vi "rethinkdb_json_paths.vi"(8 "error in (no error)":errorcluster, 10 "args":string[](array[string]), 11 "tokens":T1[](array[typedef])) -> (0 "error out":errorcluster, 2 "value_indexes":i32[](array[numeric]), 3 "value_paths":string[](array[string]), 5 "indent":i32[](array[numeric]))   [LabVIEW 2017]
uses:
  rethinkdb_json_token.ctl
panel:
  # "a -> {\"a\":1}\na/b -> {\"a\":{\"b\":1}}\na@0 -> {\"a\":[1]}\na@0/b -> {\"a\":[{\"b\":1}]"
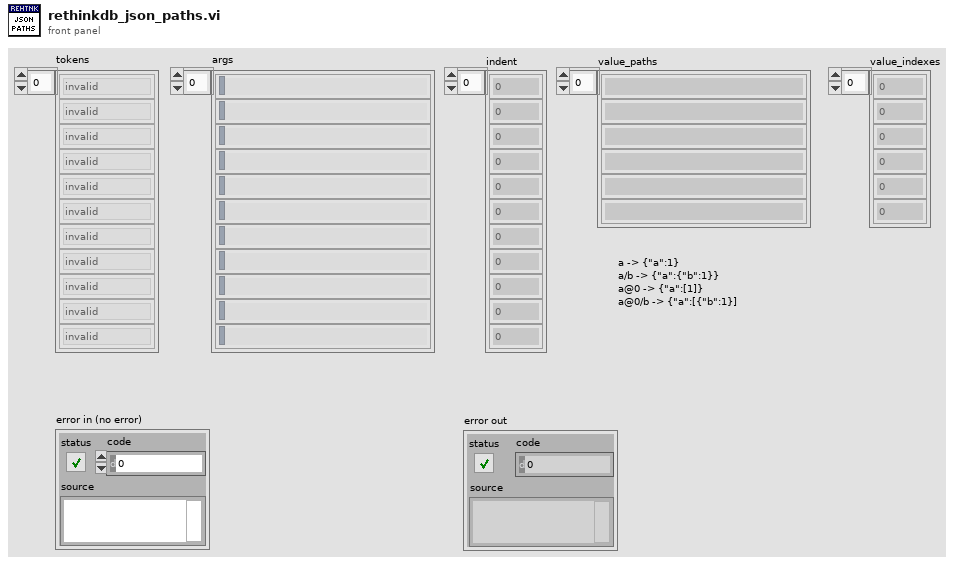
[diagram p1: front panel]
types:
  T1 = typedef "rethinkdb_json_token.ctl" = enum8{"invalid", "null", "boolean", "decimal", "float", "string", "key", "comma", "object_start", "object_end", "array_start", "array_end", "end"}
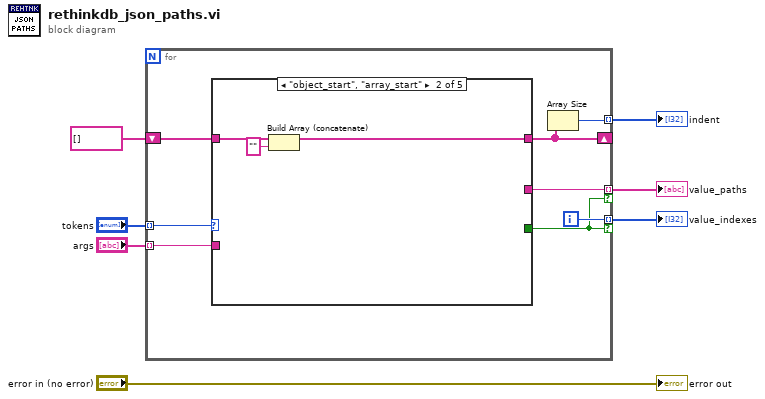
[diagram p0: block diagram]
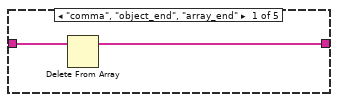
[diagram p2: hidden frame]
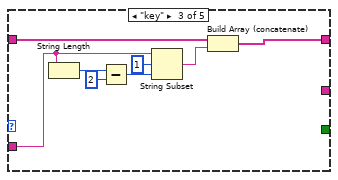
[diagram p3: hidden frame]
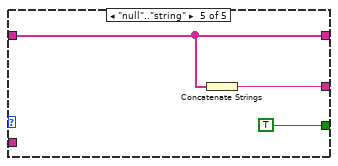
[diagram p5: hidden frame]
diagram:
  n1 = for {
    tunnel: "tokens" -> [w15] mode=indexing
    tunnel: [w12] -> w6 mode=indexing
    shift-right: [w13] -> _
    shift-left: string[] [] -> [w14]
    tunnel: "args" -> [w11] mode=indexing
    tunnel: [w10] -> w3 mode=indexing if=w8
    tunnel: [w9] -> w2 mode=indexing if=w8
    i -> [w9]
    n2 = case shown="\"object_start\", \"array_start\"" w15 {
      tunnel: [w16 w19 w27 _ w31] -> w13
      tunnel: w14 -> [w17 w20 w28 _ w31]
      tunnel: w11 -> [_ _ w22 _ _]
      tunnel: [_ _ _ _ w30] -> w10
      tunnel: [_ _ _ _ TRUE] -> w8
      frame "comma", "object_end", "array_end" {
        n3 = Delete From Array(array=w17) -> (array with subset deleted=w16:string[])  [unwired: 2 in, 1 out]
      }
      frame "object_start", "array_start" {
        n4 = Build Array (concatenate)(w20, "") -> (w19:string[])
      }
      frame "key" {
        n5 = String Length(string=w22) -> (length=w25:i32)
        n6 = Subtract(x=w25, y=2) -> (x-y=w23:i32)
        n7 = String Subset(string=w22, offset (0)=1, length (rest)=w23) -> (substring=w21:string)
        n8 = Build Array (concatenate)(w28, w21) -> (w27:string[])
      }
      frame "invalid", "end" {
      }
      frame "null".."string" {
        n9 = Concatenate Strings(w31) -> (w30:string)
      }
    }
    n10 = Array Size(array=w13) -> (size(s)=w12:i32)
  }
  "indent" <- w6
  "value_paths" <- w3
  "value_indexes" <- w2
  "error out" <- "error in (no error)"
